vi "sc_RWSerial.vi"(5 "Query?":bool, 6 "error in (no error)":errorcluster, 7 "Delay (ms)":u32=300, 8 "Command":string, 9 "VISA handle":refnum<visa-resource-name>) -> (0 "error out":errorcluster, 2 "Response":string, 3 "Dup. VISA handle":refnum<visa-resource-name>, 4 "TimeoutFlag":bool)   [LabVIEW 2019]
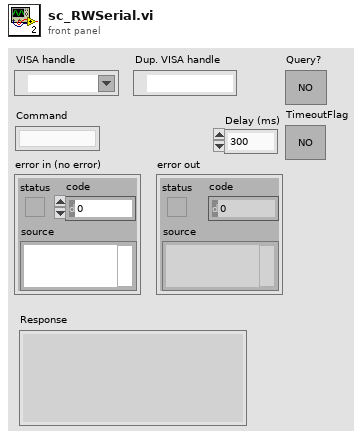
[diagram p1: front panel]
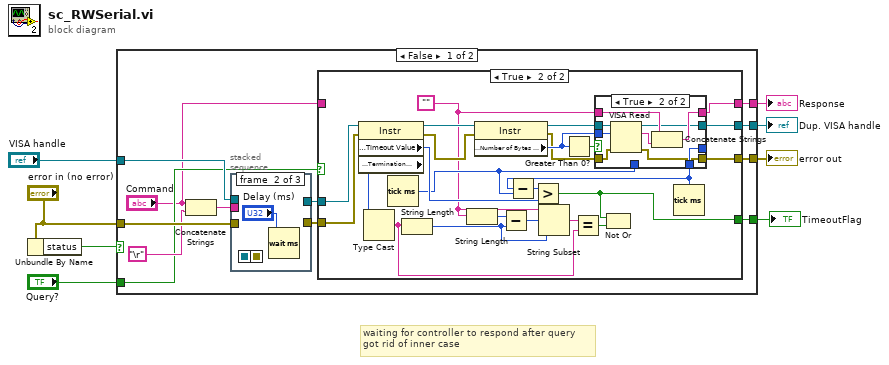
[diagram p0: block diagram]
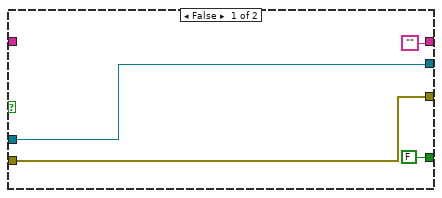
[diagram p2: hidden frame]
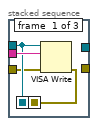
[diagram p4: hidden frame]
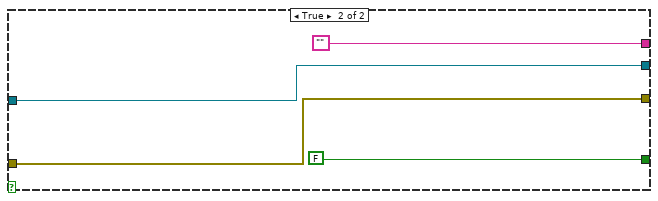
[diagram p6: hidden frame]
diagram:
  # "waiting for controller to respond after query\ngot rid of inner case"
  n1 = Unbundle By Name("error in (no error)") -> ("status"=w6:bool)
  n2 = case shown="False" w6 {
    tunnel: "VISA handle" -> [w20 w72]
    tunnel: [w16 w72] -> w8
    tunnel: [w15 w71] -> w7
    tunnel: "error in (no error)" -> [w19 w71]
    tunnel: [w14 ""] -> w4
    tunnel: [w13 FALSE] -> w3
    tunnel: "Query?" -> [w10 _]
    frame False {
      n3 = Concatenate Strings("Command", "\r") -> (w12:string)
      n4 = stacked-sequence {
        seq-local: [w64 _ _] -> [_ _ w68]
        seq-local: [w62 _ _] -> [_ _ w67]
        tunnel: w20 -> [w64 _ _]
        tunnel: w12 -> [w65 _ _]
        tunnel: w19 -> [w63 _ _]
        tunnel: [_ _ w68] -> w18
        tunnel: [_ _ w67] -> w17
        frame #0 {
          n5 = VISA Write(VISA resource name=w64, write buffer=w65, error in (no error)=w63) -> (error out=w62:errorcluster)  [unwired: 2 out]
        }
        frame #1 {
          n6 = Wait (ms)(milliseconds to wait="Delay (ms)") -> ()  [unwired: 1 out]
        }
        frame #2 {
        }
      }
      n7 = case shown="True" w10 {
        tunnel: w18 -> [w21 w48]
        tunnel: w17 -> [w22 w47]
        tunnel: [w21 w46] -> w16
        tunnel: [w22 w45] -> w15
        tunnel: ["" w44] -> w14
        tunnel: [FALSE w43] -> w13
        tunnel: "Command" -> [_ _]
        frame False {
        }
        frame True {
          w35 = ""
          n8 = property class="Instr"(reference=w48, error in=w47) -> (reference out=w42:refnum<visa-resource-name>, error out=w41:errorcluster, "General Settings:Timeout Value"=w40:u32, "Message Based Settings:Termination Character"=w38:u8)
          n9 = Type Cast(x=w38) -> (*(type *) &x=w36:string)  [unwired: 1 out]
          n10 = Tick Count (ms)() -> (millisecond timer value=w37:u32)
          n11 = String Length(string=w36) -> (length=w39:i32)
          n12 = String Length(string=w35) -> (length=w29:i32)
          n13 = property class="Instr"(reference=w42, error in=w41) -> (reference out=w33:refnum<visa-resource-name>, error out=w25:errorcluster, "Serial Settings:Number of Bytes at Serial Port"=w32:u32)
          n14 = Subtract(x=w29, y=w39) -> (x-y=w28:i32)
          n15 = String Subset(string=w35, offset (0)=w28, length (rest)=w39) -> (substring=w27:string)
          n16 = Greater Than 0?(x=w32) -> (x > 0?=w34:bool)
          n17 = Equal?(x=w27, y=w36) -> (x = y?=w26:bool)
          n18 = Tick Count (ms)() -> (millisecond timer value=w31:u32)
          n19 = Subtract(x=w31, y=w37) -> (x-y=w30:u32)
          n20 = Greater?(x=w30, y=w40) -> (0:w43:bool)
          n21 = case shown="True" w34 {
            tunnel: w33 -> [w50 w61]
            tunnel: w32 -> [_ w60]
            tunnel: w35 -> [w52 w58]
            tunnel: [w52 w57] -> w44
            tunnel: w31 -> [_ w56]
            tunnel: [w51 w56] -> _
            tunnel: w37 -> [w51 _]
            tunnel: [w50 w55] -> w46
            tunnel: w25 -> [w49 w54]
            tunnel: [w49 w53] -> w45
            frame False {
            }
            frame True {
              n22 = VISA Read(VISA resource name=w61, byte count=w60, error in (no error)=w54) -> (VISA resource name out=w55:refnum<visa-resource-name>, read buffer=w59:string, error out=w53:errorcluster)  [unwired: 1 out]
              n23 = Concatenate Strings(w58, w59) -> (w57:string)
            }
          }
          n24 = Not Or(1:w26, 2:w43) -> ()  [unwired: 1 out]
        }
      }
    }
    frame True {
    }
  }
  "Dup. VISA handle" <- w8
  "error out" <- w7
  "Response" <- w4
  "TimeoutFlag" <- w3
